vi "Read Folder.vi"(8 "error in":errorcluster, 10 "recursive?":bool, 11 "File Path":path) -> (0 "error out":errorcluster, 3 "File Paths out":path[](array[path]))   [LabVIEW 2024]
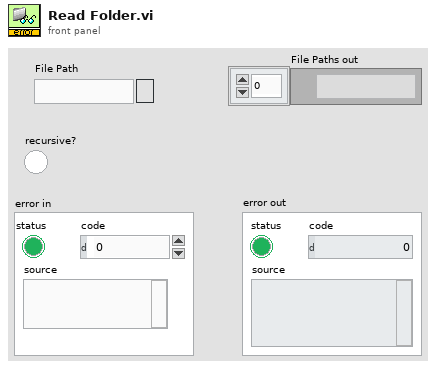
[diagram p1: front panel]
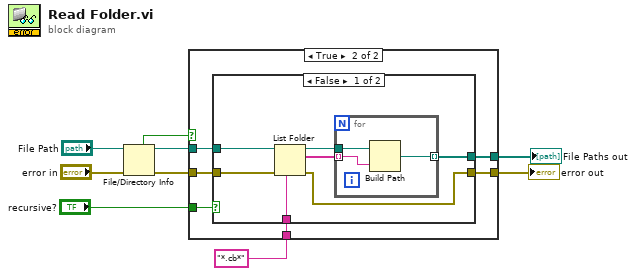
[diagram p0: block diagram]
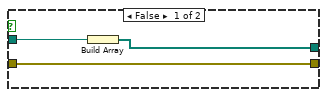
[diagram p2: hidden frame]
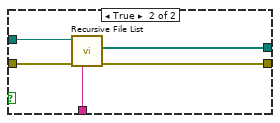
[diagram p3: hidden frame]
diagram:
  n1 = File/Directory Info(path="File Path", error in="error in") -> (path out=w7:path, directory=w6:bool, error out=w5:errorcluster)  [unwired: 4 out]
  n2 = case shown="True" w6 {
    tunnel: [w10 w18] -> w2
    tunnel: [w12 w17] -> w1
    tunnel: w5 -> [w12 w16]
    tunnel: w7 -> [w11 w15]
    tunnel: "recursive?" -> [_ w14]
    tunnel: "*.cb*" ("pattern") -> [_ w13]
    frame False {
      n3 = Build Array(w11) -> (w10:path[])
    }
    frame True {
      n4 = case shown="False" w14 {
        tunnel: [w20 w33] -> w18
        tunnel: [w19 w32] -> w17
        tunnel: w16 -> [w24 w31]
        tunnel: w15 -> [w25 w30]
        tunnel: w13 -> [w22 w29]
        frame False {
          n5 = List Folder(path=w25, pattern=w22, error in=w24) -> (path out=w21:path, filenames=w23:string[], error out=w19:errorcluster)  [unwired: 1 in, 1 out]
          n6 = for {
            tunnel: w23 -> [w28] mode=indexing
            tunnel: w21 -> [w27]
            tunnel: [w26] -> w20 mode=indexing
            n7 = Build Path(base path=w27, name or relative path=w28) -> (appended path=w26:path)
          }
        }
        frame True {
          n8 = call <vilib>:"Recursive File List.vi"("pattern"=w29, "error in (no error)"=w31, "Folder Path"=w30) -> ("error out"=w32:errorcluster, "All Files in Dir"=w33:path[])  [unwired: 4 in, 3 out]
        }
      }
    }
  }
  "File Paths out" <- w2
  "error out" <- w1
